vi "Un-Defer.vi"(8 "Error In":errorcluster, 11 "Deferer in":refnum<class "Deferer.lvclass">) -> (0 "Error Out":errorcluster)   [LabVIEW 2017, in "MGI-Panel Manager.lvlib" / "Deferer.lvclass"]
doc: "Un-defers the current instance.\n\nThe panel will only be un-deferred once ALL requesting deferrers un-defer.\n<B>Deferer In:</B> Panel Helper object to handle Defer\n<B>Error In:</B> Describes error conditions that occur before this node runs.\n\n<B>Error Out:</B> Contains error information.\n----\nPlease see the following web address for additional documentation and tutorial information:\nhttp://www.mooregoodideas.com/mgi-panel-manager/\n\nAuthor: Derek Trepanier\n\nCopyright (c) 2018, Moore Good Ideas, Inc.\n\nAll rights reserved.\n\nRedistribution and use in source and binary forms, with or without modification, are permitted provided that the following conditions are met:\n\n * Redistributions of source code must retain the above copyright notice, this list of conditions and the following disclaimer.\n * Redistributions in binary form must reproduce the above copyright notice, this list of conditions and the following disclaimer in the documentation and/or other materials provided with the distribution.\n * Neither the name of Moore Good Ideas, Inc. nor the names of its contributors may be used to endorse or promote products derived from this software without specific prior written permission.\n\nTHIS SOFTWARE IS PROVIDED BY THE COPYRIGHT HOLDERS AND CONTRIBUTORS \"AS IS\" AND ANY EXPRESS OR IMPLIED WARRANTIES, INCLUDING, BUT NOT LIMITED TO, THE IMPLIED WARRANTIES OF MERCHANTABILITY AND FITNESS FOR A PARTICULAR PURPOSE ARE DISCLAIMED. IN NO EVENT SHALL THE COPYRIGHT OWNER OR CONTRIBUTORS BE LIABLE FOR ANY DIRECT, INDIRECT, INCIDENTAL, SPECIAL, EXEMPLARY, OR CONSEQUENTIAL DAMAGES (INCLUDING, BUT NOT LIMITED TO, PROCUREMENT OF SUBSTITUTE GOODS OR SERVICES; LOSS OF USE, DATA, OR PROFITS; OR BUSINESS INTERRUPTION) HOWEVER CAUSED AND ON ANY THEORY OF LIABILITY, WHETHER IN CONTRACT, STRICT LIABILITY, OR TORT (INCLUDING NEGLIGENCE OR OTHERWISE) ARISING IN ANY WAY OUT OF THE USE OF THIS SOFTWARE, EVEN IF ADVISED OF THE POSSIBILITY OF SUCH DAMAGE."
uses:
  Deferer.lvclass
  Panel Control Counter/Panel Control Counter.lvclass
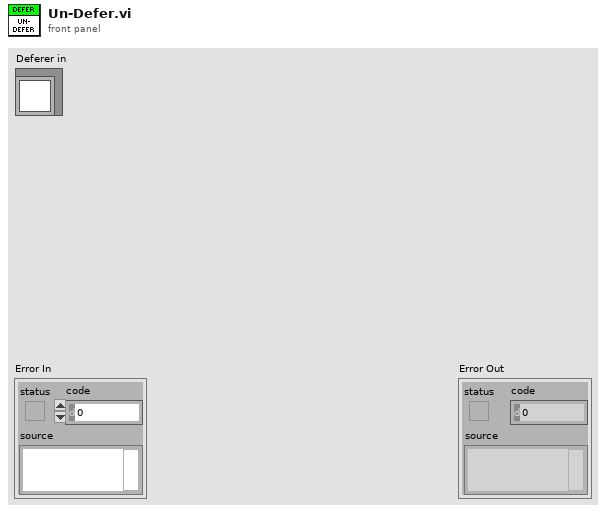
[diagram p1: front panel]
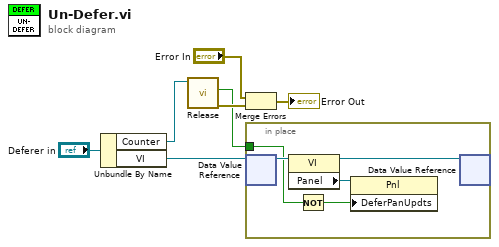
[diagram p0: block diagram]
diagram:
  n1 = Unbundle By Name("Deferer in") -> ("Counter"=w1:refnum<class "Panel Control Counter.lvclass">, "VI"=w5:refnum<data-value>)
  n2 = call "Release.vi"("Panel Control Counter in"=w1) -> ("error out"=w4:errorcluster, "Fully Released?"=w3:bool)  [unwired: 9 in]
  n3 = Merge Errors("Error In", w4) -> (→"Error Out":errorcluster)
  n4 = in-place {
    in-place-border: w3 -> [w9]
    n5 = in-place-dvr #1(w5) -> (w12:refnum<vi>)  [unwired: 1 out]
    n6 = property class="VI"(reference=w12) -> (reference out=w11:refnum<vi>, "Panel"=w10:refnum<vi>)  [unwired: 1 in, 1 out]
    n7 = Not(x=w9) -> (.not. x?=w8:bool)
    n8 = property class="Pnl"(reference=w10, "DeferPanUpdts"=w8) -> ()  [unwired: 1 in, 2 out]
    n9 = in-place-dvr #1(w11) -> ()  [unwired: 2 out]
  }
